vi "SystemInfoToKeyValuePairs.vi"(11 "system info":T2) -> (3 "hardware info key value pair":T1[](array[typedef]))   [LabVIEW 2017]
uses:
  <vilib>/addons/cRIODetectHW/control/SystemHW.ctl
  <vilib>/addons/cRIODetectHW/control/cRIO Product Info.ctl
  <vilib>/addons/InsightCM/MessageBus/Base/controls/KeyValuePair.ctl
  <vilib>/addons/cRIODetectHW/cRIODetectHW.lvlib
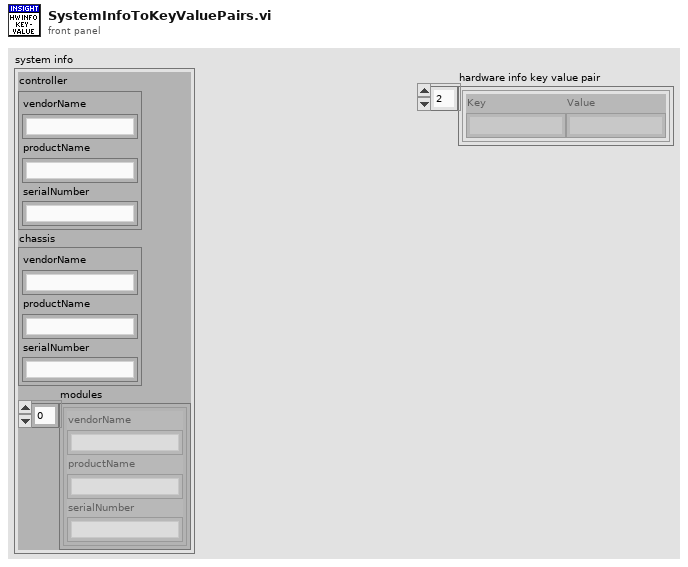
[diagram p1: front panel]
types:
  T1 = typedef "KeyValuePair.ctl" = cluster{"Key":string, "Value":string}
  T2 = typedef "cRIODetectHW.lvlib/SystemHW.ctl" = cluster{"controller":T3, "chassis":T3, "modules":T3[]}
  T3 = typedef "cRIODetectHW.lvlib/cRIO Product Info.ctl" = cluster{"vendorName":string, "productName":string, "serialNumber":string}
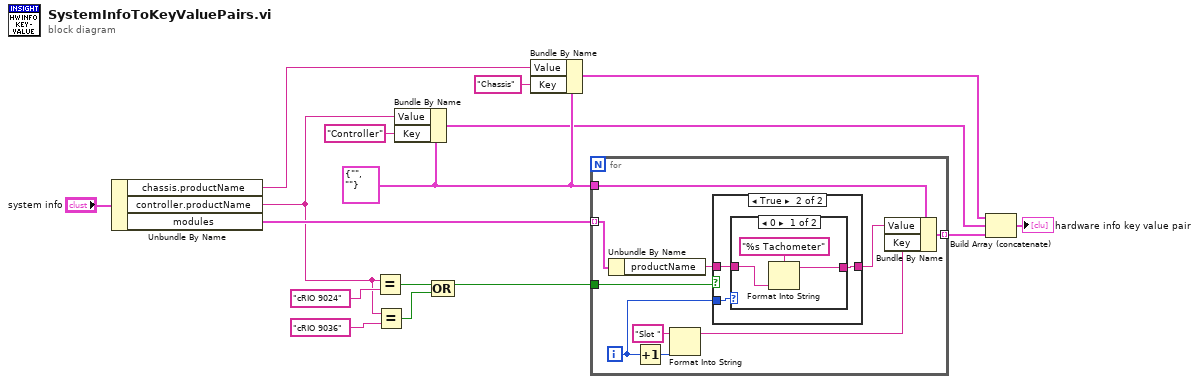
[diagram p0: block diagram]
diagram:
  w12 = T1 {"Key"="", "Value"=""}
  n1 = Unbundle By Name("system info") -> ("chassis.productName"=w10:string, "controller.productName"=w3:string, "modules"=w13:T3[])
  n2 = Equal?(x=w3, y="cRIO 9024") -> (x = y?=w5:bool)
  n3 = Equal?(x=w3, y="cRIO 9036") -> (x = y?=w1:bool)
  n4 = Bundle By Name(cluster=w12, "Value"=w3, "Key"="Controller") -> (w8:T1)
  n5 = Compound Arithmetic op=OR(w5, w1) -> (w2:bool)
  n6 = Bundle By Name(cluster=w12, "Value"=w10, "Key"="Chassis") -> (w9:T1)
  n7 = for {
    tunnel: w13 -> [w25] mode=indexing
    tunnel: w12 -> [w24]
    tunnel: [w22] -> w11 mode=indexing
    tunnel: w2 -> [w20]
    i -> [w19]
    n8 = Unbundle By Name(w25) -> ("productName"=w18:string)
    n9 = Increment(x=w19) -> (x+1=w26:i32)
    n10 = Format Into String(initial string="Slot ", w26) -> (resulting string=w21:string)  [unwired: 2 in, 1 out]
    n11 = case shown="True" w20 {
      tunnel: [w27 w30] -> w17
      tunnel: w19 -> [_ w29]
      tunnel: w18 -> [w27 w28]
      frame False {
      }
      frame True {
        n12 = case shown="0" w29 {
          tunnel: [w33 w34] -> w30
          tunnel: w28 -> [w31 w34]
          frame 0 {
            n13 = Format Into String(format string="%s Tachometer", w31) -> (resulting string=w33:string)  [unwired: 2 in, 1 out]
          }
          frame 1, Default {
          }
        }
      }
    }
    n14 = Bundle By Name(cluster=w24, "Value"=w17, "Key"=w21) -> (w22:T1)
  }
  n15 = Build Array (concatenate)(w9, w8, w11) -> (→"hardware info key value pair":T1[])
